vi "Untitled 1 (SubVI).vi"(8 "Filter ON":bool, 9 "Cluster":T1={"Parameter 1"=0.0, "Parameter 2"=0.0, "Camera view angle"=30.7} {"Camera view angle" format="%#_13g"}, 10 "Image Dst Out":T2, 11 "Refnum in":T2) -> (0 "output cluster":cluster{dbl, dbl, bool}, 1 "Distance (in)":dbl, 2 "Number of Particles":i32=1, 3 "Refnum out":T2(plugin-control))   [LabVIEW 2013]
uses:
  <vilib>/vision/Image Controls.llb/IMAQ Image.ctl
  <vilib>/vision/NI_Vision_Development_Module.lvlib
panel:
  out "Distance (in) 2":dbl
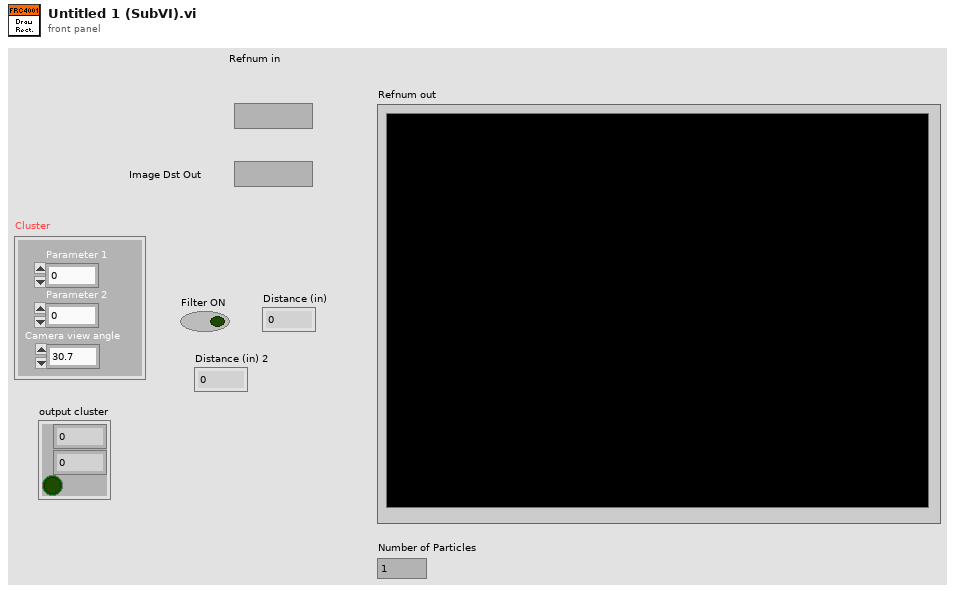
[diagram p1: front panel]
types:
  T1 = cluster{"Parameter 1":dbl, "Parameter 2":dbl, "Camera view angle":dbl}
  T2 = typedef "IMAQ Image.ctl" = refnum<image>
  T3 = typedef "Particle Parameters" = i32
  T4 = cluster{"Numeric":dbl, "Numeric":dbl, "Numeric":dbl, "Numeric":dbl}
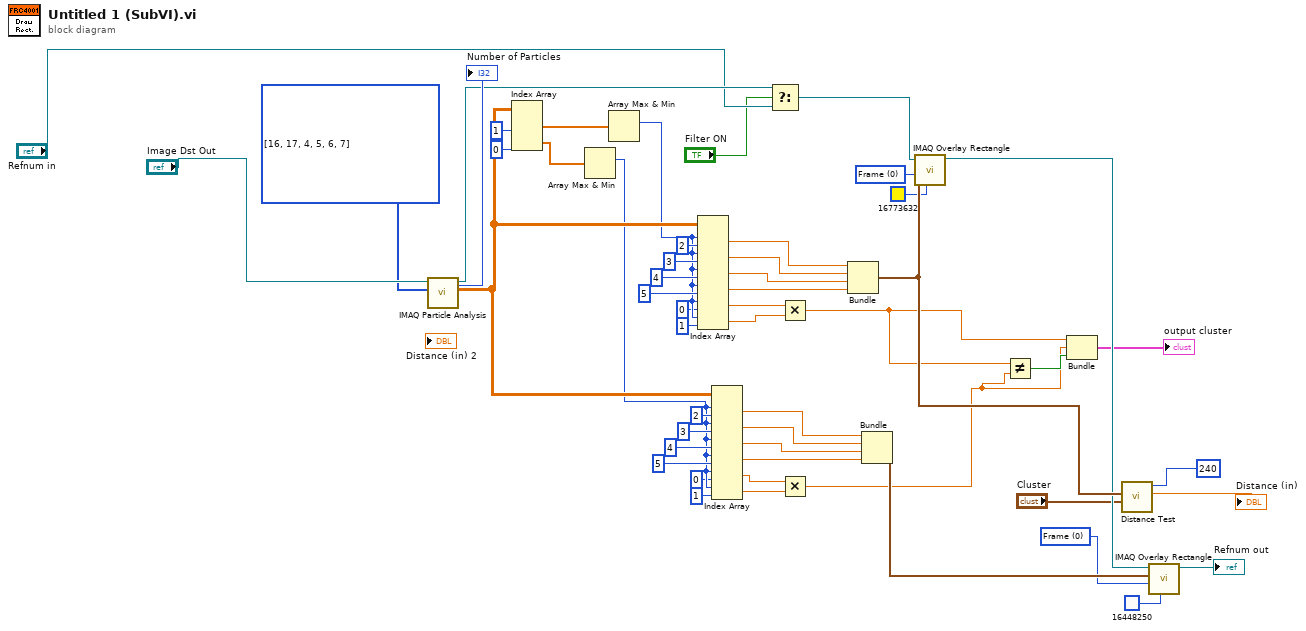
[diagram p0: block diagram]
diagram:
  w22 = u32 0 items=["Frame", "Fill", "Highlight"] ("Drawing Mode (Frame)")
  w50 = T3[] [16, 17, 4, 5, 6, 7] items=["Center of Mass X", "Center of Mass Y", "First Pixel X", "First Pixel Y", "Bounding Rect Left", "Bounding Rect Top", "Bounding Rect Right", "Bounding Rect Bottom", "Max Feret Diameter Start X", "Max Feret Diameter Start Y", "Max Feret Diameter End X", "Max Feret Diameter End Y", "Max Horiz. Segment Length Left", "Max Horiz. Segment Length Right", "Max Horiz. Segment Length Row", "-", "Bounding Rect Width", "Bounding Rect Height", "Bounding Rect Diagonal", "Perimeter", "Convex Hull Perimeter", "Holes' Perimeter", "Max Feret Diameter", "Equivalent Ellipse Major Axis", "Equivalent Ellipse Minor Axis", "Equivalent Ellipse Minor Axis (Feret)", "Equivalent Rect Long Side", "Equivalent Rect Short Side", "Equivalent Rect Diagonal", "Equivalent Rect Short Side (Feret)", "Average Horiz. Segment Length", "Average Vert. Segment Length", "Hydraulic Radius", "Waddel Disk Diameter", "-", "Area", "Holes' Area", "Particle & Holes' Area", "Convex Hull Area", "Image Area", "-", "Number of Holes", "Number of Horiz. Segments", "Number of Vert. Segments", "-", "Orientation", "Max Feret Diameter Orientation", "-", "% Area/Image Area", "% Area/(Particle & Holes' Area)", "Ratio of Equivalent Ellipse Axes", "Ratio of Equivalent Rect Sides", "-", "Elongation Factor", "Compactness Factor", "Heywood Circularity Factor", "Type Factor", "-", "Sum X", "Sum Y", "Sum XX", "Sum XY", "Sum YY", "Sum XXX", "Sum XXY", "Sum XYY", "Sum YYY", "-", "Moment of Inertia XX", "Moment of Inertia XY", "Moment of Inertia YY", "Moment of Inertia XXX", "Moment of Inertia XXY", "Moment of Inertia XYY", "Moment of Inertia YYY", "Norm. Moment of Inertia XX", "Norm. Moment of Inertia XY", "Norm. Moment of Inertia YY", "Norm. Moment of Inertia XXX", "Norm. Moment of Inertia XXY", "Norm. Moment of Inertia XYY", "Norm. Moment of Inertia YYY", "Hu Moment 1", "Hu Moment 2", "Hu Moment 3", "Hu Moment 4", "Hu Moment 5", "Hu Moment 6", "Hu Moment 7"] ("Pixel Measurements")
  w38 = u32 0 items=["Frame", "Fill", "Highlight"] ("Drawing Mode (Frame)")
  n1 = call "IMAQ Particle Analysis"("Pixel Measurements"=w50, "Image"="Image Dst Out") -> ("Particle Measurements (Pixels)"=w26:dbl[][], "Image Out (duplicate)"=w18:T2, "Number of Particles"=→"Number of Particles":i32)  [unwired: 3 in, 4 out]
  n2 = Index Array(array=w26, index (col) #1=1 ("disabled index (col)"), index (col) #2=0 ("index (col)")) -> (element #1=w21:dbl[], element #2=w20:dbl[])  [unwired: 2 in]
  n3 = Array Max & Min(array=w20) -> (max index (indices)=w9:i32)  [unwired: 3 out]
  n4 = Array Max & Min(array=w21) -> (max index (indices)=w14:i32)  [unwired: 3 out]
  n5 = Index Array(array=w26, index (row) #1=w14, index (col) #1=2 ("disabled index (col)"), index (row) #2=w14, index (col) #2=3 ("index (col)"), index (row) #3=w14, index (col) #3=4 ("index (col)"), index (row) #4=w14, index (col) #4=5 ("index (col)"), index (row) #5=w14, index (col) #5=0 ("disabled index (col)"), index (row) #6=w14, index (col) #6=1 ("disabled index (col)")) -> (element #1=w42:dbl, element #2=w43:dbl, element #3=w46:dbl, element #4=w47:dbl, element #5=w11:dbl, element #6=w10:dbl)
  n6 = Index Array(array=w26, index (row) #1=w9, index (col) #1=2 ("disabled index (col)"), index (row) #2=w9, index (col) #2=3 ("index (col)"), index (row) #3=w9, index (col) #3=4 ("index (col)"), index (row) #4=w9, index (col) #4=5 ("index (col)"), index (row) #5=w9, index (col) #5=0 ("disabled index (col)"), index (row) #6=w9, index (col) #6=1 ("disabled index (col)")) -> (element #1=w29:dbl, element #2=w30:dbl, element #3=w33:dbl, element #4=w34:dbl, element #5=w6:dbl, element #6=w5:dbl)
  n7 = Select(t=w18, s="Filter ON", f="Refnum in") -> (s? t:f=w19:T2)
  n8 = Multiply(x=w11, y=w10) -> (x*y=w2:dbl)
  n9 = Multiply(x=w6, y=w5) -> (x*y=w1:dbl)
  n10 = Bundle("Numeric"=w42, "Numeric"=w43, "Numeric"=w46, "Numeric"=w47) -> (w52:T4)  [unwired: 1 in]
  n11 = Bundle("Numeric"=w29, "Numeric"=w30, "Numeric"=w33, "Numeric"=w34) -> (w25:T4)  [unwired: 1 in]
  n12 = call "IMAQ Overlay Rectangle"("Color"=u32 16773632, "Drawing Mode (Frame)"=w38, "Rectangle"=w52, "Image"=w19) -> ("Image Out"=w24:T2)  [unwired: 6 in, 1 out]
  n13 = Not Equal?(x=w2, y=w1) -> (x != y?=w4:bool)
  n14 = Bundle(w2, w1, w4) -> (→"output cluster":cluster{dbl, dbl, bool})  [unwired: 1 in]
  n15 = call "Distance Test.vi"("Cluster"="Cluster", "Rectangle"=w52, "Y Image Resolution"=240) -> ("Distance (in)"=→"Distance (in)":dbl)  [unwired: 8 in]
  n16 = call "IMAQ Overlay Rectangle"("Color"=u32 16448250, "Drawing Mode (Frame)"=w22, "Rectangle"=w25, "Image"=w24) -> ("Image Out"=→"Refnum out":T2)  [unwired: 6 in, 1 out]
